vi "CHECK_If_TTL_should_be_reset.vi"(2 "Error In":errorcluster, 3 "To be activated in":bool[](array[boolean])) -> (0 "Error Out":errorcluster, 1 "To be activated out":bool[](array[boolean]))   [LabVIEW 2018, in "Tracker.lvlib"]
uses:
  Tracker.lvlib
  <vilib>/ptbypt/NI_PtbyPt.lvlib
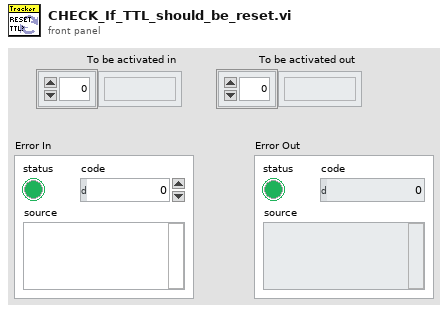
[diagram p1: front panel]
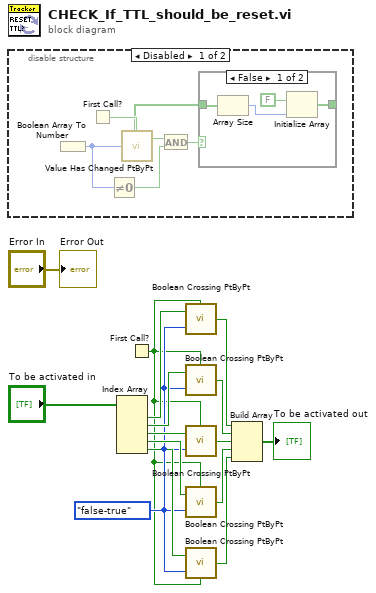
[diagram p0: block diagram]
diagram:
  w3 = enum16{"either", "false-true", "true-false"}."false-true" ("direction")
  n1 = disable-structure shown="Disabled" {
    frame Disabled {
      n2 = First Call?() -> (First Call?: T/F=w21:bool)
      n3 = Boolean Array To Number(Boolean array=w16) -> (number=w20:u32)
      n4 = Not Equal To 0?(x=w20) -> (x != 0?=w19:bool)
      n5 = call <vilib>:"Value Has Changed PtByPt.vi"("input data point"=w20, "initialize"=w21) -> ("has changed"=w18:bool)  [unwired: 1 out]
      n6 = And(x=w18, y=w19) -> (x .and. y?=w17:bool)
      n7 = case shown="False" w17 {
        tunnel: [w22 w26] -> _
        tunnel: [w25 w26] -> w16
        frame False {
          n8 = Array Size(array=w25) -> (size(s)=w24:i32)
          n9 = Initialize Array(FALSE, w24) -> (w22:bool[])
        }
        frame True {
        }
      }
    }
    frame Enabled {
    }
  }
  n10 = Index Array(array="To be activated in") -> (element #1=w14:bool, element #2=w13:bool, element #3=w12:bool, element #4=w11:bool, element #5=w4:bool)  [unwired: 5 in]
  n11 = First Call?() -> (First Call?: T/F=w2:bool)
  n12 = call <vilib>:"Boolean Crossing PtByPt.vi"("initialize"=w2, "direction"=w3, "input"=w14) -> ("crossing"=w10:bool)
  n13 = call <vilib>:"Boolean Crossing PtByPt.vi"("initialize"=w2, "direction"=w3, "input"=w13) -> ("crossing"=w9:bool)
  n14 = call <vilib>:"Boolean Crossing PtByPt.vi"("initialize"=w2, "direction"=w3, "input"=w12) -> ("crossing"=w8:bool)
  n15 = call <vilib>:"Boolean Crossing PtByPt.vi"("initialize"=w2, "direction"=w3, "input"=w11) -> ("crossing"=w7:bool)
  n16 = call <vilib>:"Boolean Crossing PtByPt.vi"("initialize"=w2, "direction"=w3, "input"=w4) -> ("crossing"=w1:bool)
  n17 = Build Array(w10, w9, w8, w7, w1) -> (→"To be activated out":bool[])
  "Error Out" <- "Error In"
